vi "Configure Group.vi"(0 "VISA resource name":refnum<visa-resource-name>, 1 "Channel (no array)":string[](array[string]), 5 "Group Number (1)":i32=1 min=1 max=60 step=1, 7 "Enable Group (False)":bool, 9 "Group Name (\"\")":string, 11 "error in (no error)":errorcluster) -> (4 "VISA resource name out":refnum<visa-resource-name>, 6 "Group Number":i32, 15 "error out":errorcluster)   [LabVIEW 2020, in "Yokogawa GX Series.lvlib"]
doc: "Sets the group.\n\nCommand: SGroup"
uses:
  <instrlib>/Yokogawa GX Series/Yokogawa GX Series.lvlib
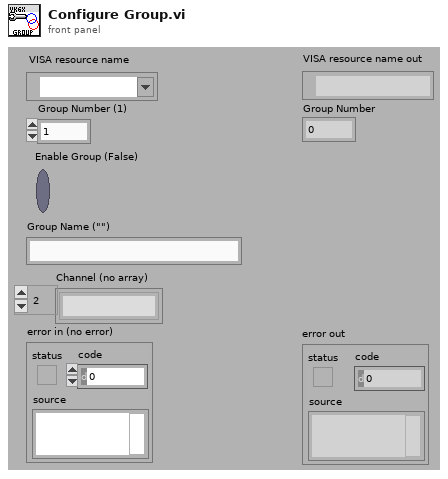
[diagram p1: front panel]
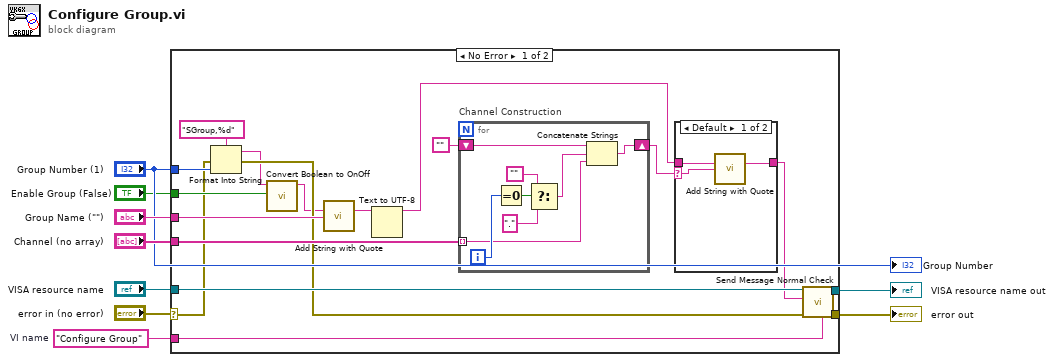
[diagram p0: block diagram]
diagram:
  w8 = "Configure Group"  # VI name
  n1 = case shown="No Error" "error in (no error)" {
    selector: "error in (no error)" -> [w12 w40]
    tunnel: "Channel (no array)" -> [w26 _]
    tunnel: w8 -> [w25 _]
    tunnel: [w24 w41] -> w7
    tunnel: [w23 w40] -> w6
    tunnel: "VISA resource name" -> [w22 w41]
    tunnel: "Group Name (\"\")" -> [w21 _]
    tunnel: "Group Number (1)" -> [w18 _]
    tunnel: "Enable Group (False)" -> [w16 _]
    frame No Error {
      n2 = Format Into String(format string="SGroup,%d", error in=w12, w18) -> (resulting string=w17:string, error out=w19:errorcluster)  [unwired: 1 in]
      n3 = call <instrlib>:"Convert Boolean to OnOff.vi"("On/Off"=w16, "Initial String (\"\")"=w17) -> ("Resulting String"=w15:string)  [unwired: 9 in]
      n4 = call <instrlib>:"Add String with Quote.vi"("Initial String (\"\")"=w15, "String (\"\")"=w21) -> ("Resulting String"=w11:string)  [unwired: 12 in, 1 out]
      n5 = Text to UTF-8(11:w11) -> (3:w10:string)  [unwired: 2 in, 1 out]
      n6 = for "Channel Construction" {
        tunnel: w26 -> [w32] mode=indexing
        shift-right: [w38] -> w14
        shift-left: "" -> [w39]
        i -> [w37]
        n7 = Equal To 0?(x=w37) -> (x = 0?=w36:bool)
        n8 = Select(t="", s=w36, f=".") -> (s? t:f=w35:string)
        n9 = Concatenate Strings(w39, w35, w32) -> (w38:string)
      }
      n10 = case shown="Default" w14 {
        selector: w14 -> [w30 _]
        tunnel: [w29 w31] -> w13
        tunnel: w10 -> [w28 w31]
        frame Default {
          n11 = call <instrlib>:"Add String with Quote.vi"("Initial String (\"\")"=w28, "String (\"\")"=w30) -> ("Resulting String"=w29:string)  [unwired: 12 in, 1 out]
        }
        frame "" {
        }
      }
      n12 = call <instrlib>:"Send Message Normal Check.vi"("Source (\"\")"=w25, "error in (no error)"=w19, "Send Message (\"\")"=w13, "VISA resource name"=w22) -> ("error out"=w23:errorcluster, "VISA resource name out"=w24:refnum<visa-resource-name>)  [unwired: 2 in, 4 out]
    }
    frame Error {
    }
  }
  "error out" <- w6
  "VISA resource name out" <- w7
  "Group Number" <- "Group Number (1)"
